vi "Pass If Equal.vi"(6 "Delta":variant, 7 "Description":string, 8 "error in (no error)":errorcluster, 9 "Actual":variant, 10 "Expected":variant, 11 "LUnit Test Case In":refnum<class "LUnit Inheriting Test Case.lvclass">) -> (0 "error out":errorcluster, 3 "LUnit Test Case Out":refnum<class "LUnit Inheriting Test Case.lvclass">)   [LabVIEW 2020]
doc: "***DEPRECATED*** Use the maleable (.vim) version of this VI instead. \n\nGenerates a pass result for the calling test method if the inputs are equal. For numeric inputs, a tolerance range may be specified using the Delta input. A description may be provided to the result."
uses:
  cbf50e99-f124-4847-863a-8e9794d3dede.vi
  LUnit Inheriting Test Case.lvclass
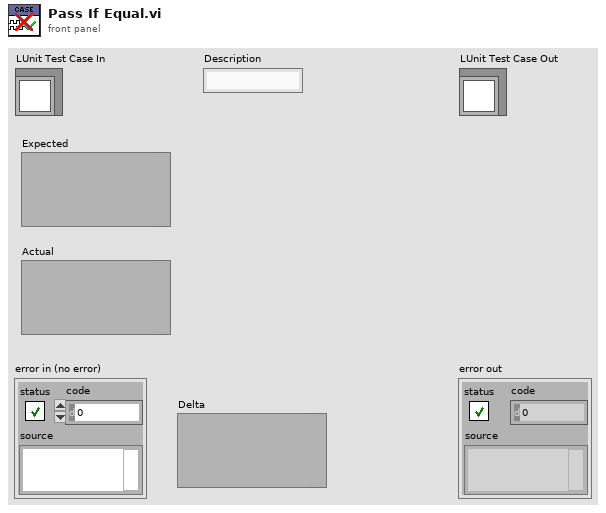
[diagram p1: front panel]
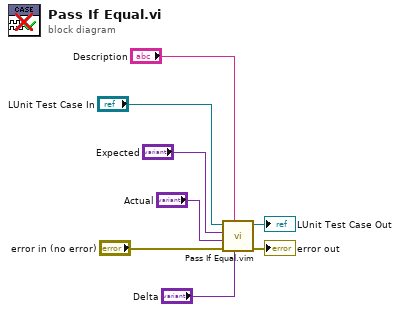
[diagram p0: block diagram]
diagram:
  n1 = call "Pass If Equal.vim"("Delta"="Delta", "Description"="Description", "error in (no error)"="error in (no error)", "Actual"="Actual", "Expected"="Expected", "LUnit Test Case In"="LUnit Test Case In") -> ("error out"=→"error out":errorcluster, "LUnit Test Case Out"=→"LUnit Test Case Out":refnum<class "LUnit Inheriting Test Case.lvclass">)  [unwired: 4 in]
